vi "ShooterStateMachine.vi"(6 "Shooter Delay (ms)":u32=1500, 9 "Encoder Distance":dbl=1400.0, 10 "Retract Timeout":u32=5000, 11 "Winch Speed":dbl=-1.0) -> ()   [LabVIEW 2013]
doc: "State machine to manage the shooter related functions."
uses:
  ShooterStates.ctl
  ShooterCmds.ctl
  <vilib>/Rock Robotics/WPI/Solenoid/WPI_SolenoidValue.ctl
  <vilib>/Rock Robotics/WPI/Solenoid/WPI_SolenoidSetEnum.vi
panel:
  in  "Auto \nShooter Delay (ms)":u32=750
  in  "Release Timeout":u32=5000
  in  "Release Speed":dbl=0.5
  in  "Clutch Delay (ms)":u32=100
  in  "Full Encoder Distance":dbl
  in  "Retract Full Timeout":u32=5000
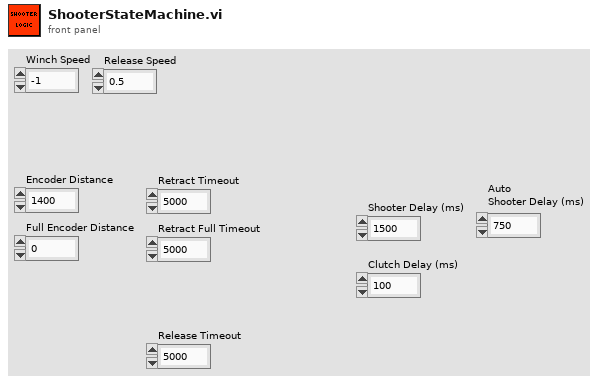
[diagram p1: front panel]
types:
  T1 = cluster{"Fire After Retract Full ":bool, "Full Reset":bool, "Reset After Fire":bool, "Auto":bool, "Zeroed":bool}
  T2 = typedef "ShooterCmds.ctl" = enum16{"Fire", "Lob", "Retract", "End Of Match", "Release", "FireAuto"}
  T3 = typedef "ShooterStates.ctl" = enum16{"Init", "Ready", "RetractFull", "Disengage Clutch", "Clutch Delay", "Fire", "Fire Delay", "Latch", "Retract", "Release"}
  T4 = typedef "WPI_DigitalInputDevRef.ctl" = cluster{"DevStatus":errorcluster, "DIO Channel":T5, "Digital Module":T6}
  T5 = typedef "FPGA_DIOChannel.ctl" = enum8{"DIO 1", "DIO 2", "DIO 3", "DIO 4", "DIO 5", "DIO 6", "DIO 7", "DIO 8", "DIO 9", "DIO 10", "DIO 11", "DIO 12", "DIO 13", "DIO 14", "Invalid"}
  T6 = typedef "FPGA_TypedefDigitalModule.ctl" = enum16{"Digital Module 1", "Digital Module 2"}
  T7 = typedef "WPI_EncoderDevRef.ctl" = cluster{"DevStatus":errorcluster, "EncoderIndex":T8, "CounterIndex":T9, "DistancePerCount":dbl, "Decoding Type":T10}
  T8 = typedef "FPGA_EncoderIdx.ctl" = enum8{"Enc 0", "Enc 1", "Enc 2", "Enc 3", "Invalid"}
  T9 = typedef "FPGA_CounterCtrSystemIndex.ctl" = enum8{"Ctr 0", "Ctr 1", "Ctr 2", "Ctr 3", "Ctr 4", "Ctr 5", "Ctr 6", "Ctr 7", "Invalid"}
  T10 = typedef "WPI_EncoderType.ctl" = enum16{"1x", "2x", "4x"}
  T11 = typedef "WPI_SolenoidDevRef.ctl" = cluster{"DevStatus":errorcluster, "Solenoid Module":T12, "Forward Solenoid Channel":T13, "Reverse Solenoid Channel":T13}
  T12 = typedef "FPGA_TypedefSolenoidModule.ctl" = enum16{"Solenoid Module 1", "Solenoid Module 2"}
  T13 = typedef "WPI_SolenoidChannel.ctl" = enum8{"Solenoid 1", "Solenoid 2", "Solenoid 3", "Solenoid 4", "Solenoid 5", "Solenoid 6", "Solenoid 7", "Solenoid 8", "Invalid"}
  T14 = typedef "WPI_MotorControlDeviceRef.ctl" = cluster{"DeviceStatus":errorcluster, "Type":enum16{"PWM", "CAN"}, "PWM":cluster{"Digital Module":T6, "PWM Channel":T15, "DeadBand":T16}, "CAN":cluster{"Device Number":u8, "Control Mode":T17, "Semaphore":T18, "Max Vout":dbl}, "Invert":bool, "TransformRef":T19, "InvTransformRef":T19}
  T15 = typedef "FPGA_DIOPWMChannel.ctl" = enum8{"PWM 1", "PWM 2", "PWM 3", "PWM 4", "PWM 5", "PWM 6", "PWM 7", "PWM 8", "PWM 9", "PWM 10", "Invalid"}
  T16 = typedef "WPI_PWMDeadband.ctl" = cluster{"Name":string, "maxPositivePwm":i32, "minPositivePwm":i32, "centerPwm":i32, "maxNegativePwm":i32, "minNegativePwm":i32, "angularRange":u16}
  T17 = typedef "WPI_CANJaguar_ControlMode.ctl" = enum8{"Percent VBus", "Current", "Speed", "Position", "Voltage"}
  T18 = typedef "Semaphore RefNum" = refnum<k1>
  T19 = typedef "WPI_PWMTransform_ConPane.ctl" = refnum<vi>
  T20 = cluster{"Shooter Ratchet":T11, "Shooter Limit":T4, "Shooter Dog":T11, "Wipers":T11, "Winch":T14, "Encoder":T7}
  T21 = typedef "WPI_SolenoidValue.ctl" = enum16{"Off", "On", "Forward", "Reverse"}
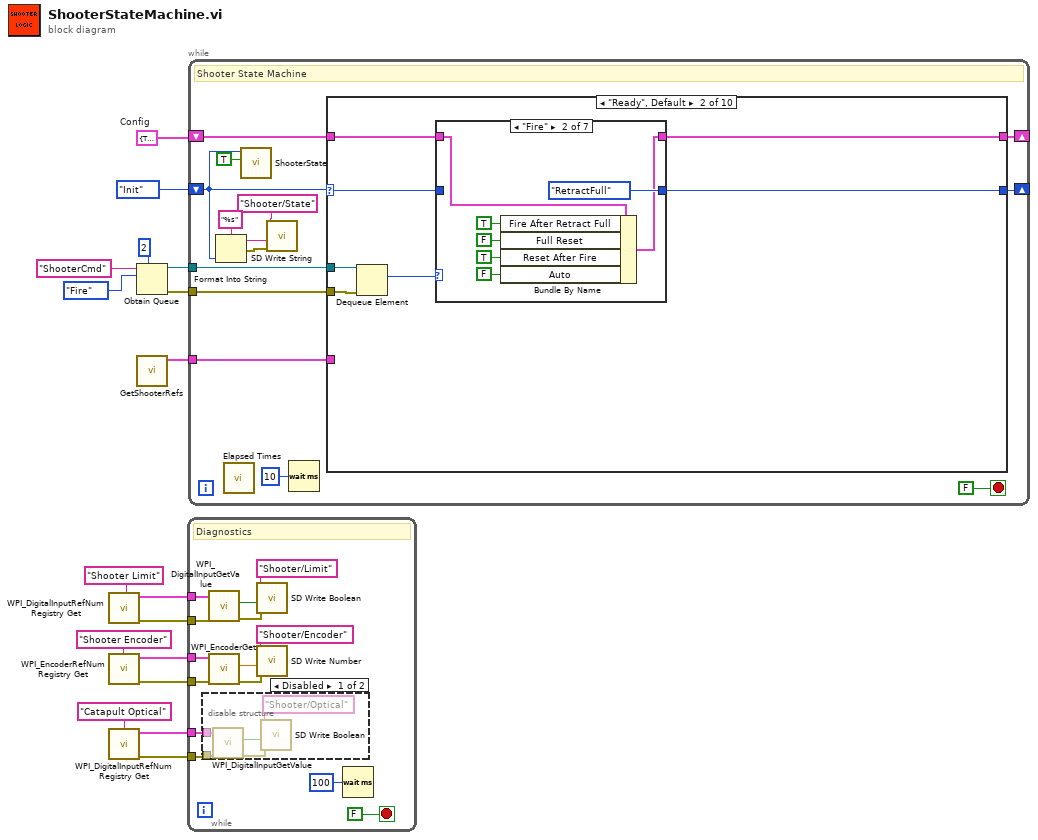
[diagram p0: block diagram]
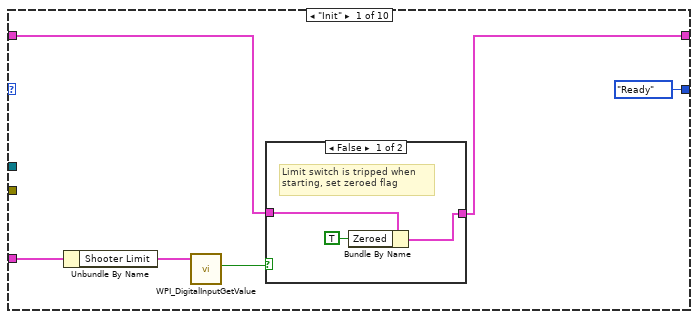
[diagram p2: hidden frame]
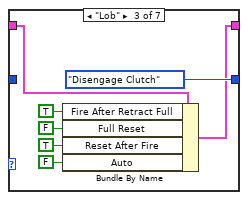
[diagram p5: hidden frame]
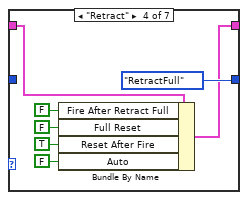
[diagram p6: hidden frame]
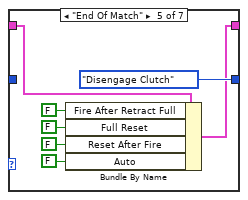
[diagram p7: hidden frame]
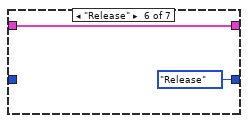
[diagram p8: hidden frame]
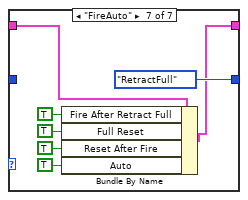
[diagram p9: hidden frame]
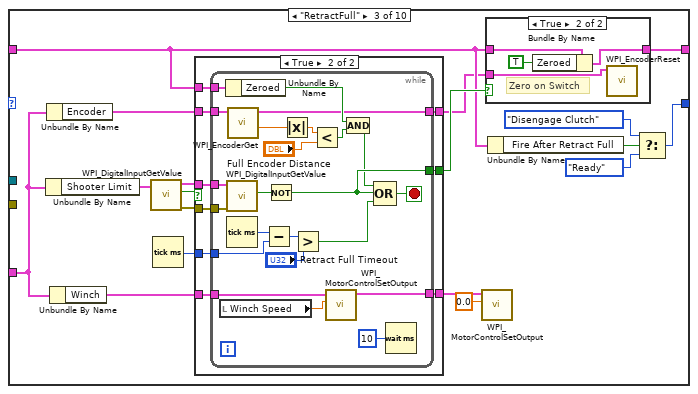
[diagram p10: hidden frame]
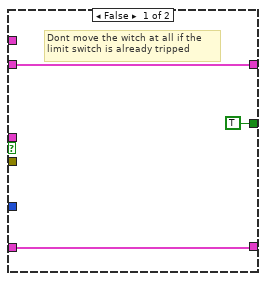
[diagram p12: hidden frame]
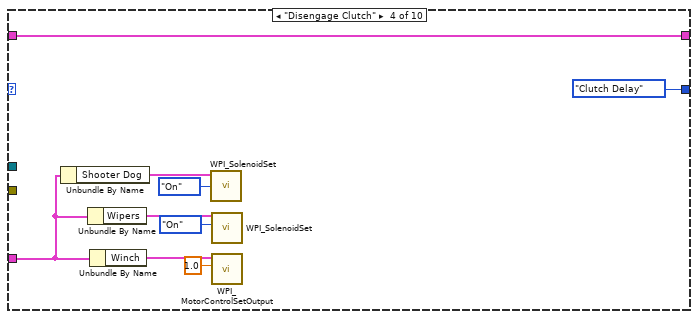
[diagram p13: hidden frame]
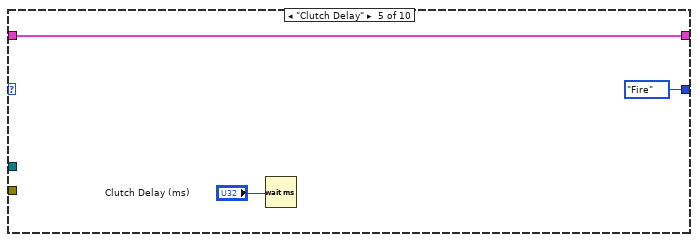
[diagram p14: hidden frame]
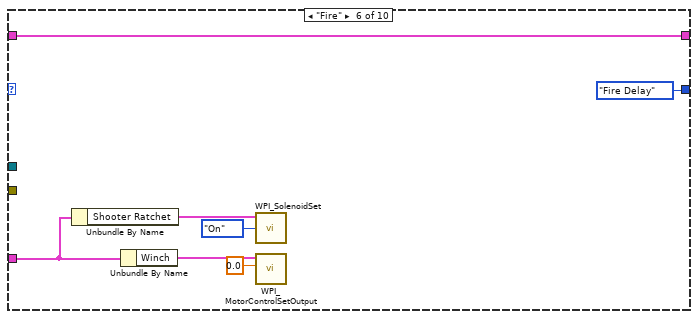
[diagram p15: hidden frame]
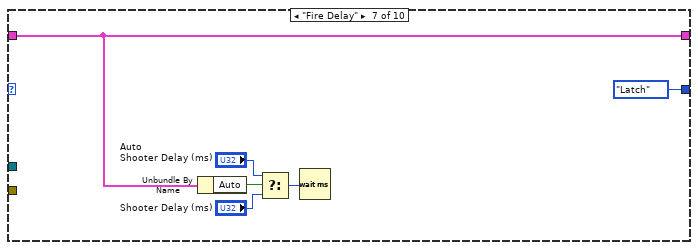
[diagram p16: hidden frame]
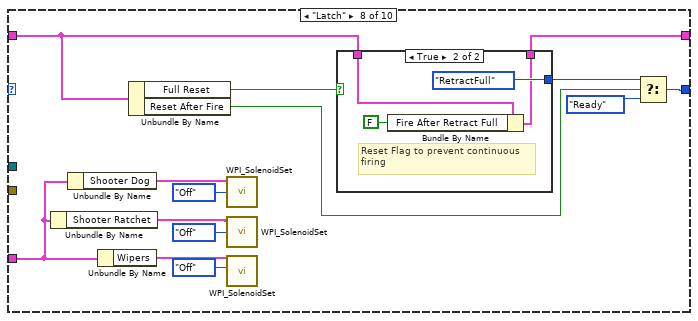
[diagram p17: hidden frame]
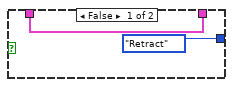
[diagram p18: hidden frame]
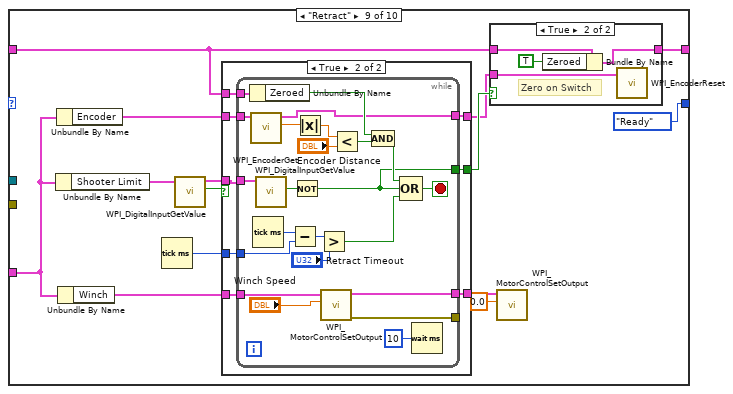
[diagram p19: hidden frame]
diagram:
  w1 = T1 {"Fire After Retract Full "=TRUE, "Full Reset"=FALSE, "Reset After Fire"=TRUE, "Auto"=FALSE, "Zeroed"=FALSE}  # Config
  n1 = call <vilib>:"WPI_DigitalInputRefNum Registry Get.vi"("refnum name"="Shooter Limit") -> ("error out"=w14:errorcluster, "DigitalInputDevRef"=w15:T4)  [unwired: 9 in]
  n2 = call <vilib>:"WPI_EncoderRefNum Registry Get.vi"("refnum name"="Shooter Encoder") -> ("error out"=w12:errorcluster, "EncoderDevRef"=w13:T7)  [unwired: 9 in]
  n3 = call <vilib>:"WPI_DigitalInputRefNum Registry Get.vi"("refnum name"="Catapult Optical") -> ("error out"=w9:errorcluster, "DigitalInputDevRef"=w10:T4)  [unwired: 9 in]
  n4 = Obtain Queue(max queue size (-1, unlimited)=2, name (unnamed)="ShooterCmd", element data type=ShooterCmds."Fire") -> (queue out=w7:refnum<queue>, error out=w8:errorcluster)  [unwired: 2 in, 1 out]
  n5 = call "GetShooterRefs.vi"() -> ("cluster out"=w2:T20)  [unwired: 10 in, 1 out]
  n6 = while {
    tunnel: w15 -> [w24]
    tunnel: w14 -> [w23]
    tunnel: w13 -> [w22]
    tunnel: w12 -> [w21]
    tunnel: w10 -> [w20]
    tunnel: w9 -> [w19]
    stop <- FALSE stop-if-true
    # "Diagnostics"
    n7 = disable-structure shown="Disabled" {
      disable-tunnel: w20 -> [w33 _]
      disable-tunnel: w19 -> [w32 _]
      frame Disabled {
        n8 = call <vilib>:"WPI_DigitalInputGetValue.vi"("error in (no error)"=w32, "DigitalInputDevRef"=w33) -> ("error out"=w36:errorcluster, "Value"=w34:bool)  [unwired: 7 in, 1 out]
        n9 = call <vilib>:"SD Write Boolean.vi"("error in"=w36, "Boolean"=w34, "Name"="Shooter/Optical") -> ()  [unwired: 7 in, 2 out]
      }
      frame Enabled {
      }
    }
    n10 = call <vilib>:"WPI_DigitalInputGetValue.vi"("error in (no error)"=w23, "DigitalInputDevRef"=w24) -> ("error out"=w28:errorcluster, "Value"=w18:bool)  [unwired: 7 in, 1 out]
    n11 = call <vilib>:"WPI_EncoderGet.vi"("error in (no error)"=w21, "EncoderDevRef"=w22) -> ("error out"=w30:errorcluster, "Distance"=w29:dbl)  [unwired: 4 in, 4 out]
    n12 = call <vilib>:"SD Write Boolean.vi"("error in"=w28, "Boolean"=w18, "Name"="Shooter/Limit") -> ()  [unwired: 7 in, 2 out]
    n13 = call <vilib>:"SD Write Number.vi"("error in"=w30, "Numeric"=w29, "Name"="Shooter/Encoder") -> ()  [unwired: 7 in, 2 out]
    n14 = Wait (ms)(milliseconds to wait=u32 100) -> ()  [unwired: 1 out]
  }
  n15 = while {
    shift-right: [w47] -> _
    shift-left: ShooterStates."Init" -> [w40]
    tunnel: w7 -> [w49]
    tunnel: w8 -> [w48]
    tunnel: w2 -> [w39]
    shift-right: [w37] -> _
    shift-left: w1 -> [w38]
    stop <- FALSE stop-if-true
    # "Shooter State Machine"
    n16 = Format Into String(format string="%s", w40) -> (resulting string=w44:string, error out=w45:errorcluster)  [unwired: 2 in]
    n17 = call "Elapsed Times.vi"() -> ()  [unwired: 3 in, 1 out]
    n18 = call "ShooterState.vi"("Set?"=TRUE, "Value in"=w40) -> ()  [unwired: 9 in, 1 out]
    n19 = call <vilib>:"SD Write String.vi"("error in"=w45, "String"=w44, "Name"="Shooter/State") -> ()  [unwired: 7 in, 2 out]
    n20 = Wait (ms)(milliseconds to wait=u32 10) -> ()  [unwired: 1 out]
    n21 = case shown="\"Ready\", Default" w40 {
      selector: w40 -> [_ w64 _ _ _ _ _ _ _ _]
      tunnel: w49 -> [_ w67 _ _ _ _ _ _ _ _]
      tunnel: w48 -> [_ w66 _ _ _ _ _ _ _ _]
      tunnel: [ShooterStates."Ready" w63 w121 ShooterStates."Clutch Delay" ShooterStates."Fire" ShooterStates."Fire Delay" ShooterStates."Latch" w200 ShooterStates."Ready" ShooterStates."Ready"] -> w47
      tunnel: w39 -> [w55 _ w112 w167 _ w179 _ w194 w219 w264]
      tunnel: w38 -> [w52 w62 w109 w165 w174 w177 w184 w191 w211 w263]
      tunnel: [w51 w61 w108 w165 w174 w177 w184 w190 w212 w263] -> w37
      frame "Init" {
        n22 = Unbundle By Name(w55) -> ("Shooter Limit"=w54:T4)
        n23 = call <vilib>:"WPI_DigitalInputGetValue.vi"("DigitalInputDevRef"=w54) -> ("Value"=w53:bool)  [unwired: 8 in, 2 out]
        n24 = case shown="False" w53 {
          tunnel: w52 -> [w59 w60]
          tunnel: [w57 w60] -> w51
          frame False {
            # "Limit switch is tripped when \nstarting, set zeroed flag"
            n25 = Bundle By Name(cluster=w59, "Zeroed"=TRUE) -> (w57:T1)
          }
          frame True {
          }
        }
      }
      frame "Ready", Default {
        n26 = Dequeue Element(queue=w67, error in (no error)=w66) -> (element=w65:T2)  [unwired: 1 in, 3 out]
        n27 = case shown="\"Fire\"" w65 {
          tunnel: w64 -> [w69 _ _ _ _ _ _]
          tunnel: [w69 ShooterStates."RetractFull" ShooterStates."Disengage Clutch" ShooterStates."RetractFull" ShooterStates."Disengage Clutch" ShooterStates."Release" ShooterStates."RetractFull"] -> w63
          tunnel: w62 -> [w68 w75 w77 w85 w92 w98 w101]
          tunnel: [w68 w74 w78 w84 w91 w98 w100] -> w61
          frame Default {
            # "Unknown Command, do nothing"
          }
          frame "Fire" {
            n28 = Bundle By Name(cluster=w75, "Fire After Retract Full"=TRUE, "Full Reset"=FALSE, "Reset After Fire"=TRUE, "Auto"=FALSE) -> (w74:T1)
          }
          frame "Lob" {
            n29 = Bundle By Name(cluster=w77, "Fire After Retract Full"=TRUE, "Full Reset"=FALSE, "Reset After Fire"=TRUE, "Auto"=FALSE) -> (w78:T1)
          }
          frame "Retract" {
            n30 = Bundle By Name(cluster=w85, "Fire After Retract Full"=FALSE, "Full Reset"=FALSE, "Reset After Fire"=TRUE, "Auto"=FALSE) -> (w84:T1)
          }
          frame "End Of Match" {
            n31 = Bundle By Name(cluster=w92, "Fire After Retract Full"=FALSE, "Full Reset"=FALSE, "Reset After Fire"=FALSE, "Auto"=FALSE) -> (w91:T1)
          }
          frame "Release" {
          }
          frame "FireAuto" {
            n32 = Bundle By Name(cluster=w101, "Fire After Retract Full"=TRUE, "Full Reset"=TRUE, "Reset After Fire"=TRUE, "Auto"=TRUE) -> (w100:T1)
          }
        }
      }
      frame "RetractFull" {
        n33 = Unbundle By Name(w112) -> ("Shooter Limit"=w115:T4)
        n34 = Unbundle By Name(w112) -> ("Encoder"=w111:T7)
        n35 = Unbundle By Name(w112) -> ("Winch"=w114:T14)
        n36 = call <vilib>:"WPI_DigitalInputGetValue.vi"("DigitalInputDevRef"=w115) -> ("error out"=w117:errorcluster, "Value"=w116:bool, "DigitalInputDevRef"=w118:T4)  [unwired: 8 in]
        n37 = Tick Count (ms)() -> (millisecond timer value=w124:u32)
        n38 = case shown="True" w116 {
          tunnel: w124 -> [_ w141]
          tunnel: w114 -> [w131 w140]
          tunnel: [w131 w139] -> w123
          tunnel: [TRUE w138] -> w110
          tunnel: w118 -> [_ w137]
          tunnel: w117 -> [_ w136]
          tunnel: w109 -> [_ w135]
          tunnel: w111 -> [w130 w134]
          tunnel: [w130 w133] -> w107
          frame False {
            # "Dont move the witch at all if the \nlimit switch is already tripped"
          }
          frame True {
            n39 = while {
              tunnel: w137 -> [w164]
              tunnel: w136 -> [w163]
              tunnel: w141 -> [w160]
              tunnel: w140 -> [w155]
              tunnel: [w154] -> w139
              tunnel: [w151] -> w138
              tunnel: w135 -> [w150]
              tunnel: w134 -> [w143]
              tunnel: [w142] -> w133
              stop <- w162 stop-if-true
              n40 = local read "Winch Speed"() -> (w153:dbl)
              n41 = Unbundle By Name(w150) -> ("Zeroed"=w149:bool)
              n42 = call <vilib>:"WPI_DigitalInputGetValue.vi"("error in (no error)"=w163, "DigitalInputDevRef"=w164) -> ("Value"=w152:bool)  [unwired: 7 in, 2 out]
              n43 = Tick Count (ms)() -> (millisecond timer value=w161:u32)
              n44 = call <vilib>:"WPI_EncoderGet.vi"("EncoderDevRef"=w143) -> ("Distance"=w146:dbl, "EncoderDevRef"=w142:T7)  [unwired: 5 in, 4 out]
              n45 = Subtract(x=w161, y=w160) -> (x-y=w159:u32)
              n46 = Not(x=w152) -> (.not. x?=w151:bool)
              n47 = Absolute Value(x=w146) -> (abs(x)=w147:dbl)
              n48 = Greater?(x=w159, y="Retract Full Timeout") -> (0:w157:bool)
              n49 = Less?(x=w147, y="Full Encoder Distance") -> (x < y?=w145:bool)
              n50 = call <vilib>:"WPI_MotorControlSetOutput.vi"("Output"=w153, "MotorControlDevRef"=w155) -> ("MotorControlDevRef"=w154:T14)  [unwired: 7 in, 2 out]
              n51 = Compound Arithmetic op=AND(w149, w145) -> (w144:bool)
              n52 = Compound Arithmetic op=OR(w144, w151, w157) -> (w162:bool)
              n53 = Wait (ms)(milliseconds to wait=u32 10) -> ()  [unwired: 1 out]
            }
          }
        }
        n54 = call <vilib>:"WPI_MotorControlSetOutput.vi"("Output"=0.0, "MotorControlDevRef"=w123) -> ()  [unwired: 7 in, 3 out]
        n55 = case shown="True" w110 {
          tunnel: w109 -> [w125 w129]
          tunnel: [w125 w128] -> w108
          tunnel: w107 -> [_ w126]
          frame False {
          }
          frame True {
            # "Zero on Switch"
            n56 = Bundle By Name(cluster=w129, "Zeroed"=TRUE) -> (w128:T1)
            n57 = call <vilib>:"WPI_EncoderReset.vi"("EncoderDevRef"=w126) -> ()  [unwired: 9 in, 2 out]
          }
        }
        n58 = Unbundle By Name(w109) -> ("Fire After Retract Full"=w113:bool)
        n59 = Select(t=ShooterStates."Disengage Clutch", s=w113, f=ShooterStates."Ready") -> (s? t:f=w121:T3)
      }
      frame "Disengage Clutch" {
        n60 = Unbundle By Name(w167) -> ("Shooter Dog"=w169:T11)
        n61 = Unbundle By Name(w167) -> ("Wipers"=w168:T11)
        n62 = Unbundle By Name(w167) -> ("Winch"=w166:T14)
        n63 = call-poly <vilib>:"WPI_SolenoidSet.vi"("Value"=WPI_SolenoidValue."On", "SolenoidDevRef"=w169) -> ()  [unwired: 8 in, 2 out]
        n64 = call-poly <vilib>:"WPI_SolenoidSet.vi"("Value"=WPI_SolenoidValue."On", "SolenoidDevRef"=w168) -> ()  [unwired: 8 in, 2 out]
        n65 = call <vilib>:"WPI_MotorControlSetOutput.vi"("Output"=1.0, "MotorControlDevRef"=w166) -> ()  [unwired: 7 in, 3 out]
      }
      frame "Clutch Delay" {
        n66 = Wait (ms)(milliseconds to wait="Clutch Delay (ms)") -> ()  [unwired: 1 out]
      }
      frame "Fire" {
        n67 = Unbundle By Name(w179) -> ("Shooter Ratchet"=w180:T11)
        n68 = Unbundle By Name(w179) -> ("Winch"=w178:T14)
        n69 = call-poly <vilib>:"WPI_SolenoidSet.vi"("Value"=WPI_SolenoidValue."On", "SolenoidDevRef"=w180) -> ()  [unwired: 8 in, 2 out]
        n70 = call <vilib>:"WPI_MotorControlSetOutput.vi"("Output"=0.0, "MotorControlDevRef"=w178) -> ()  [unwired: 7 in, 3 out]
      }
      frame "Fire Delay" {
        n71 = Unbundle By Name(w184) -> ("Auto"=w185:bool)
        n72 = Select(t="Auto \nShooter Delay (ms)", s=w185, f="Shooter Delay (ms)") -> (s? t:f=w186:u32)
        n73 = Wait (ms)(milliseconds to wait=w186) -> ()  [unwired: 1 out]
      }
      frame "Latch" {
        n74 = Unbundle By Name(w194) -> ("Shooter Ratchet"=w196:T11)
        n75 = Unbundle By Name(w194) -> ("Shooter Dog"=w197:T11)
        n76 = Unbundle By Name(w194) -> ("Wipers"=w195:T11)
        n77 = Unbundle By Name(w191) -> ("Full Reset"=w193:bool, "Reset After Fire"=w192:bool)
        n78 = call-poly <vilib>:"WPI_SolenoidSet.vi"("Value"=WPI_SolenoidValue."Off", "SolenoidDevRef"=w197) -> ()  [unwired: 8 in, 2 out]
        n79 = call-poly <vilib>:"WPI_SolenoidSet.vi"("Value"=WPI_SolenoidValue."Off", "SolenoidDevRef"=w196) -> ()  [unwired: 8 in, 2 out]
        n80 = call-poly <vilib>:"WPI_SolenoidSet.vi"("Value"=WPI_SolenoidValue."Off", "SolenoidDevRef"=w195) -> ()  [unwired: 8 in, 2 out]
        n81 = case shown="True" w193 {
          tunnel: [ShooterStates."Retract" ShooterStates."RetractFull"] -> w198
          tunnel: w191 -> [w204 w208]
          tunnel: [w204 w207] -> w190
          frame False {
          }
          frame True {
            # "Reset Flag to prevent continuous\nfiring"
            n82 = Bundle By Name(cluster=w208, "Fire After Retract Full"=FALSE) -> (w207:T1)
          }
        }
        n83 = Select(t=w198, s=w192, f=ShooterStates."Ready") -> (s? t:f=w200:T3)
      }
      frame "Retract" {
        n84 = Unbundle By Name(w219) -> ("Shooter Limit"=w216:T4)
        n85 = Unbundle By Name(w219) -> ("Encoder"=w214:T7)
        n86 = Unbundle By Name(w219) -> ("Winch"=w215:T14)
        n87 = Tick Count (ms)() -> (millisecond timer value=w223:u32)
        n88 = call <vilib>:"WPI_DigitalInputGetValue.vi"("DigitalInputDevRef"=w216) -> ("Value"=w218:bool, "DigitalInputDevRef"=w217:T4)  [unwired: 8 in, 1 out]
        n89 = case shown="True" w218 {
          tunnel: w223 -> [_ w239]
          tunnel: [w230 w238] -> w222
          tunnel: w217 -> [_ w237]
          tunnel: w215 -> [w230 w236]
          tunnel: w211 -> [_ w235]
          tunnel: w214 -> [w229 w234]
          tunnel: [TRUE w233] -> w213
          tunnel: [w229 w232] -> w210
          frame False {
          }
          frame True {
            n90 = while {
              tunnel: w237 -> [w262]
              tunnel: w239 -> [w259]
              tunnel: w236 -> [w254]
              tunnel: [w253] -> w238
              tunnel: [w250] -> _
              tunnel: w235 -> [w249]
              tunnel: w234 -> [w243]
              tunnel: [w241] -> w233
              tunnel: [w240] -> w232
              stop <- w261 stop-if-true
              n91 = Unbundle By Name(w249) -> ("Zeroed"=w248:bool)
              n92 = call <vilib>:"WPI_EncoderGet.vi"("EncoderDevRef"=w243) -> ("Distance"=w242:dbl, "EncoderDevRef"=w240:T7)  [unwired: 5 in, 4 out]
              n93 = Tick Count (ms)() -> (millisecond timer value=w260:u32)
              n94 = call <vilib>:"WPI_DigitalInputGetValue.vi"("DigitalInputDevRef"=w262) -> ("Value"=w252:bool)  [unwired: 8 in, 2 out]
              n95 = Subtract(x=w260, y=w259) -> (x-y=w258:u32)
              n96 = Not(x=w252) -> (.not. x?=w241:bool)
              n97 = Absolute Value(x=w242) -> (abs(x)=w245:dbl)
              n98 = Greater?(x=w258, y="Retract Timeout") -> (0:w256:bool)
              n99 = call <vilib>:"WPI_MotorControlSetOutput.vi"("Output"="Winch Speed", "MotorControlDevRef"=w254) -> ("error out"=w250:errorcluster, "MotorControlDevRef"=w253:T14)  [unwired: 7 in, 1 out]
              n100 = Less?(x=w245, y="Encoder Distance") -> (x < y?=w244:bool)
              n101 = Compound Arithmetic op=AND(w248, w244) -> (w247:bool)
              n102 = Compound Arithmetic op=OR(w247, w241, w256) -> (w261:bool)
              n103 = Wait (ms)(milliseconds to wait=u32 10) -> ()  [unwired: 1 out]
            }
          }
        }
        n104 = case shown="True" w213 {
          tunnel: [w224 w227] -> w212
          tunnel: w211 -> [w224 w226]
          tunnel: w210 -> [_ w225]
          frame False {
          }
          frame True {
            # "Zero on Switch"
            n105 = Bundle By Name(cluster=w226, "Zeroed"=TRUE) -> (w227:T1)
            n106 = call <vilib>:"WPI_EncoderReset.vi"("EncoderDevRef"=w225) -> ()  [unwired: 9 in, 2 out]
          }
        }
        n107 = call <vilib>:"WPI_MotorControlSetOutput.vi"("Output"=0.0, "MotorControlDevRef"=w222) -> ()  [unwired: 7 in, 3 out]
      }
      frame "Release" {
        n108 = Unbundle By Name(w264) -> ("Shooter Ratchet"=w266:T11)
        n109 = Unbundle By Name(w264) -> ("Encoder"=w267:T7)
        n110 = Unbundle By Name(w264) -> ("Winch"=w265:T14)
        n111 = call-poly <vilib>:"WPI_SolenoidSet.vi"("Value"=WPI_SolenoidValue."On", "SolenoidDevRef"=w266) -> ("SolenoidDevRef"=w269:T11)  [unwired: 8 in, 1 out]
        n112 = Tick Count (ms)() -> (millisecond timer value=w275:u32)
        n113 = while {
          tunnel: w267 -> [w290]
          tunnel: w275 -> [w287]
          tunnel: w265 -> [w282]
          tunnel: [w281] -> w274
          tunnel: w269 -> [w277]
          tunnel: [w277] -> w268
          stop <- w291 stop-if-true
          n114 = local read "Encoder Distance"() -> (w278:dbl)
          n115 = Tick Count (ms)() -> (millisecond timer value=w288:u32)
          n116 = call <vilib>:"WPI_EncoderGet.vi"("EncoderDevRef"=w290) -> ("Distance"=w276:dbl)  [unwired: 5 in, 5 out]
          n117 = Subtract(x=w288, y=w287) -> (x-y=w286:u32)
          n118 = Greater?(x=w286, y="Release Timeout") -> (0:w284:bool)
          n119 = call <vilib>:"WPI_MotorControlSetOutput.vi"("Output"="Release Speed", "MotorControlDevRef"=w282) -> ("MotorControlDevRef"=w281:T14)  [unwired: 7 in, 2 out]
          n120 = Absolute Value(x=w276) -> (abs(x)=w279:dbl)
          n121 = Greater?(x=w279, y=w278) -> (0:w289:bool)
          n122 = Compound Arithmetic op=OR(w289, w284) -> (w291:bool)
          n123 = Wait (ms)(milliseconds to wait=u32 10) -> ()  [unwired: 1 out]
        }
        n124 = call <vilib>:"WPI_MotorControlSetOutput.vi"("Output"=0.0, "MotorControlDevRef"=w274) -> ()  [unwired: 7 in, 3 out]
        n125 = call-poly <vilib>:"WPI_SolenoidSet.vi"("Value"=WPI_SolenoidValue."Off", "SolenoidDevRef"=w268) -> ()  [unwired: 8 in, 2 out]
      }
    }
  }
